vi "myRIO_BRig_Host_formatData_test3_p2.vi"(7 "input_headers":string[](array[string]), 8 "input_error":errorcluster, 9 "input_Iexist":bool, 10 "input_filePath":path, 11 "input_hdl_Workbooks":refnum<k7>) -> (0 "output_error":errorcluster, 2 "output_newFilePath":path, 3 "output_hdl_Worksbooks":refnum<k7>)   [LabVIEW 2014]
uses:
  <vilib>/Utility/file.llb/Read From Spreadsheet File (I64).vi
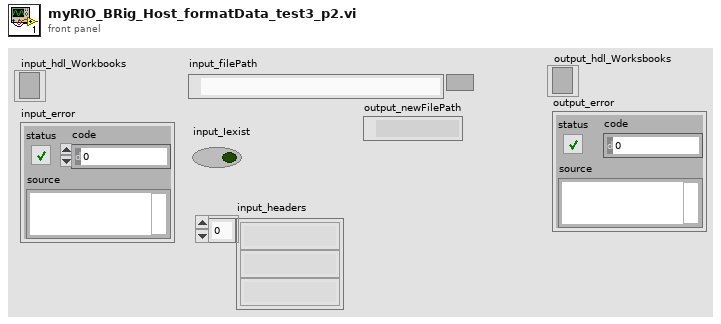
[diagram p1: front panel]
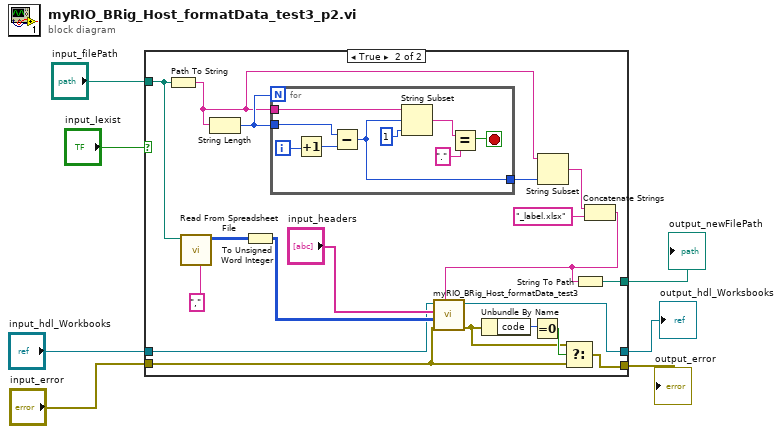
[diagram p0: block diagram]
diagram:
  n1 = case shown="True" "input_Iexist" {
    tunnel: "input_hdl_Workbooks" -> [w9 w19]
    tunnel: "input_error" -> [w8 w11]
    tunnel: [w9 w18] -> w3
    tunnel: [w8 w10] -> w2
    tunnel: "input_filePath" -> [_ w17]
    tunnel: [_ w15] -> w1
    frame False {
    }
    frame True {
      n2 = Path To String(path=w17) -> (string=w26:string)
      n3 = call-poly <vilib>:"Read From Spreadsheet File.vi"("delimiter (\\t)"="," ("delimiter (\\t)"), "file path (dialog if empty)"=w17) -> ("all rows"=w22:i64[][])  [unwired: 5 in, 4 out]
      n4 = String Length(string=w26) -> (length=w28:i32)
      n5 = To Unsigned Word Integer(number=w22) -> (unsigned 16bit integer=w21:u16[][])
      n6 = for {
        N: w28 -> [_]
        tunnel: w28 -> [w35]
        tunnel: w26 -> [w34]
        tunnel: [w29] -> w27
        i -> [w37]
        stop <- w30 stop-if-true
        n7 = Increment(x=w37) -> (x+1=w36:i32)
        n8 = Subtract(x=w35, y=w36) -> (x-y=w29:i32)
        n9 = String Subset(string=w34, offset (0)=w29, length (rest)=1 ("length (rest)")) -> (substring=w32:string)
        n10 = Equal?(x=w32, y=".") -> (x = y?=w30:bool)
      }
      n11 = String Subset(string=w26, length (rest)=w27) -> (substring=w25:string)  [unwired: 1 in]
      n12 = Concatenate Strings(w25, "_label.xlsx" ("string")) -> (w16:string)
      n13 = call "myRIO_BRig_Host_formatData_test3.vi"("input_filePath"=w16, "input_error"=w11, "input_data"=w21, "input_headers"="input_headers", "input_hdl_Workbooks"=w19) -> ("output_error"=w12:errorcluster, "output_hdl_Worksbooks"=w18:refnum<k7>)  [unwired: 5 in]
      n14 = Unbundle By Name(w12) -> ("code"=w14:i32)
      n15 = Equal To 0?(x=w14) -> (x = 0?=w13:bool)
      n16 = Select(t=w12, s=w13, f=w11) -> (s? t:f=w10:errorcluster)
      n17 = String To Path(string=w16) -> (path=w15:path)
    }
  }
  "output_hdl_Worksbooks" <- w3
  "output_error" <- w2
  "output_newFilePath" <- w1
